vi "VARIANT.vi"() -> ()   [LabVIEW 2022 SP3]
panel:
  out "names":string[](array[string])
  in  "INFO":string[](array[string])
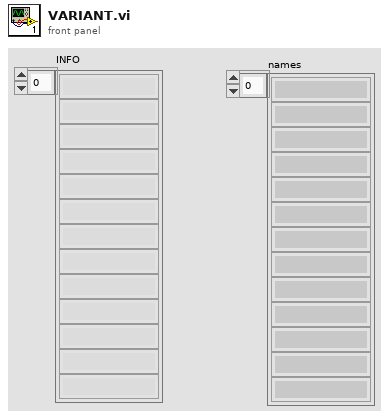
[diagram p1: front panel]
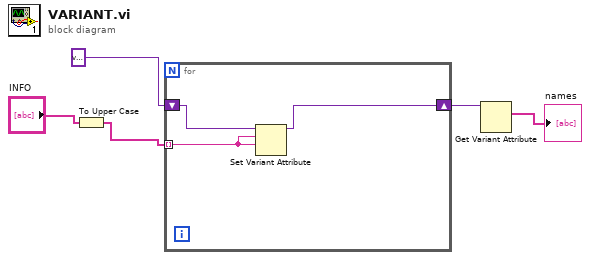
[diagram p0: block diagram]
diagram:
  n1 = To Upper Case(1:"INFO") -> (0:w4:string[])
  n2 = for {
    tunnel: w4 -> [w6] mode=indexing
    shift-right: [w7] -> w2
    shift-left: variant -> [w8]
    n3 = Set Variant Attribute(Variant=w8, name=w6, value=w6) -> (Variant out=w7:variant)  [unwired: 1 in, 2 out]
  }
  n4 = Get Variant Attribute(Variant=w2) -> (names=→"names":string[])  [unwired: 3 in, 3 out]
